vi "Close MeasurementLink Session.vi"(8 "error in":errorcluster, 9 "initialize and close session behavior":T1, 10 "session in":variant, 11 "session factory in":refnum<class "Session Factory.lvclass">) -> (0 "error out":errorcluster)   [LabVIEW 2021, in "Session Management niDAQmx.lvlib" / "Session Factory.lvclass"]
doc: "Closes the local session. If the session represents a remote session, <b>initialize and close session behavior</b> determines whether closing the local session closes the server session or detaches from the server session."
uses:
  Session Factory.lvclass
  <vilib>/Plug-In SDKs/Sessions/Instrument/ISession Factory/Initialize and Close Session Behavior.ctl
  Session Factory.lvclass/Session Factory.ctl
  Client/NI_DAQmx_client/RPC Messages/nidaqmx_grpc_ClearTaskRequest.ctl
  Client/NI_DAQmx_client/RPC Messages/nidevice_grpc_Session.ctl
  Client/NI_DAQmx_client/RPC Messages/nidevice_grpc_Session_session/nidevice_grpc_Session_session.lvclass
  Client/NI_DAQmx_client/NI_DAQmx_client.lvlib
  <vilib>/Plug-In SDKs/Sessions/Instrument/ISession Factory/ISession Factory.lvclass
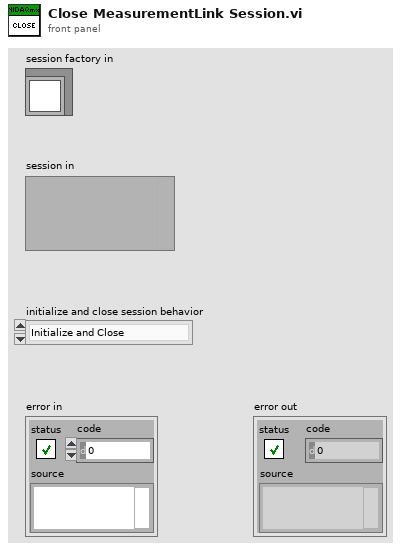
[diagram p1: front panel]
types:
  T1 = typedef "NI Session Management Instrument.lvlib/ISession Factory.lvclass/Initialize and Close Session Behavior.ctl" = enum16{"Initialize and Close", "Attach and Detach", "Initialize and Detach", "Attach and Close"}
  T2 = typedef "NI_DAQmx_client.lvlib/nidaqmx_grpc_ClearTaskRequest.ctl" = cluster{"task":T3}
  T3 = typedef "NI_DAQmx_client.lvlib/nidevice_grpc_Session.ctl" = cluster{"nidevice_grpc_Session_session":refnum<class "nidevice_grpc_Session_session.lvclass">}
  T4 = typedef "grpc-lvsupport-release.lvlib/grpcId.ctl" = u64
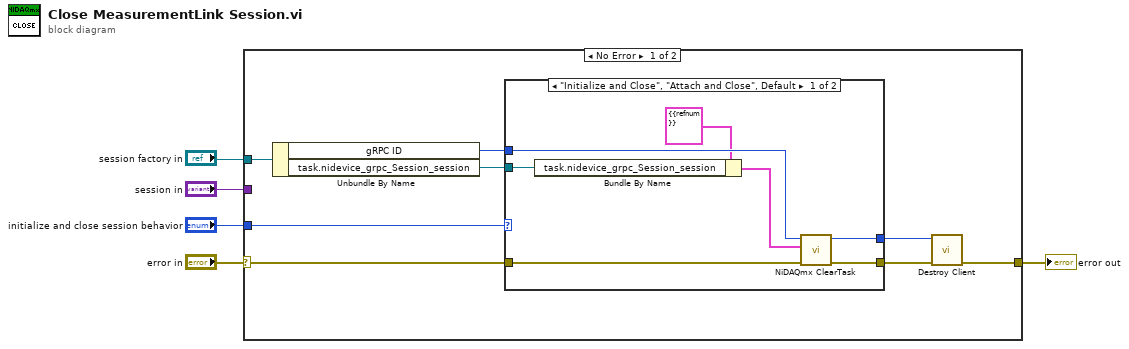
[diagram p0: block diagram]
diagram:
  n1 = case shown="No Error" "error in" {
    selector: "error in" -> [w12 w23]
    tunnel: [w6 w23] -> w4
    tunnel: "session factory in" -> [w13 _]
    tunnel: "session in" -> [_ _]
    tunnel: "initialize and close session behavior" -> [w9 _]
    frame No Error {
      n2 = Unbundle By Name(w13) -> ("gRPC ID"=w11:T4, "task.nidevice_grpc_Session_session"=w10:refnum<class "nidevice_grpc_Session_session.lvclass">)
      n3 = case shown="\"Initialize and Close\", \"Attach and Close\", Default" w9 {
        tunnel: w12 -> [w20 w21]
        tunnel: [w19 w21] -> w7
        tunnel: w11 -> [w18 w22]
        tunnel: w10 -> [w16 _]
        tunnel: [w14 w22] -> w8
        frame "Initialize and Close", "Attach and Close", Default {
          n4 = Bundle By Name(cluster=T2 {"task"={"nidevice_grpc_Session_session"=refnum}} ("Request Data"), "task.nidevice_grpc_Session_session"=w16) -> (w15:T2)
          n5 = call "NiDAQmx ClearTask.vi"("error in"=w20, "Request Data"=w15, "gRPC ID"=w18) -> ("error out"=w19:errorcluster, "gRPC ID out"=w14:T4)  [unwired: 6 in, 1 out]
        }
        frame "Attach and Detach", "Initialize and Detach" {
        }
      }
      n6 = call "Destroy Client.vi"("error in"=w7, "gRPC ID"=w8) -> ("error out"=w6:errorcluster)  [unwired: 9 in]
    }
    frame Error {
    }
  }
  "error out" <- w4
